vi "ConnectBlueTooth.vi"(0 "NXT name":string="Sasha Al", 1 "Connection type":T2) -> (2 "NXTObject":T1 {"nxtIterHandle" format="%08x"; "modIterHandle" format="%08x"; "moduleHandle" format="%08x"; "fileIterHandle" format="%08x"; "fileHandle" format="%08x"; "nxtHandle" format="%08x"}, 3 "Is Paired with NXT?":bool, 4 "error out":errorcluster)   [LabVIEW 2011]
uses:
  <vilib>/NXT/NXT Controls/ConnectionType.ctl
  <vilib>/NXT/Block Support/nxt.ctl
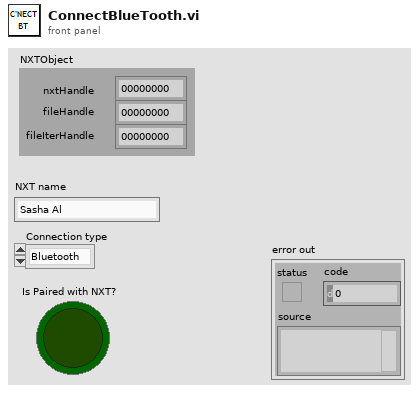
[diagram p1: front panel]
types:
  T1 = typedef "nxt.ctl" = cluster{"nxtHandle":u32, "fileHandle":u32, "fileIterHandle":u32, "moduleHandle":u32, "modIterHandle":u32, "nxtIterHandle":u32}
  T2 = typedef "ConnectionType.ctl" = enum16{"Bluetooth", "USB", "WiFi"}
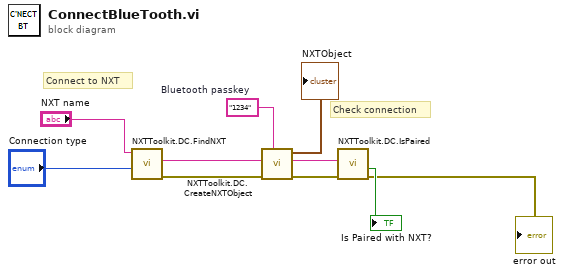
[diagram p0: block diagram]
diagram:
  w11 = "1234"  # Bluetooth passkey
  # "Check connection"
  # "Connect to NXT"
  n1 = call <vilib>:"NXTToolkit.DC.FindNXT.vi"("Connection type (USB)"="Connection type", "NXT name"="NXT name") -> ("error out"=w10:errorcluster, "VISA resource string"=w9:string)  [unwired: 7 in, 1 out]
  n2 = call <vilib>:"NXTToolkit.DC.CreateNXTObject.vi"("Bluetooth passkey (1234)"=w11, "error in (no error)"=w10, "VISA resource string (\"\" : find USB brick)"=w9) -> ("error out"=w8:errorcluster, "VISA resource string out"=w7:string, "NXTObject"=→"NXTObject":T1)  [unwired: 6 in]
  n3 = call <vilib>:"NXTToolkit.DC.IsPaired.vi"("error in (no error)"=w8, "VISA resource string"=w7) -> ("error out"=→"error out":errorcluster, "Is Paired?"=→"Is Paired with NXT?":bool, "VISA resource string dup"=w3:string)  [unwired: 7 in]
